vi "Start.vi"(8 "error in (no error)":errorcluster, 10 "Message in":refnum<class "StartMessage.lvclass">, 11 "ImageStack in":refnum<class "Invivo_ImageStack.lvclass">) -> (0 "error out":errorcluster, 3 "ImageStack out":refnum<class "Invivo_ImageStack.lvclass">)   [LabVIEW 2012, in "Invivo_ImageStack.lvclass"]
doc: "This member function is called when the statemachine in the run.vi receives an 'start' command. It relays the message to all observers of the component.\n\nOverride this member function in your derived class if you need additional start functionality (but don't forget to call the parent method)."
uses:
  Invivo_ImageStack.lvclass
  <vilib>/Distrio/Murmex/StartMessage/StartMessage.lvclass
  <vilib>/Distrio/Murmex/StartMessage/run mode enum.ctl
  <vilib>/Distrio/Murmex/GenericMessage/GenericMessage.lvclass
  Invivo_ImageStack.lvclass/Invivo_ImageStack.ctl
  <vilib>/Distrio/Murmex/Murmex/Murmex.lvclass
  <vilib>/Distrio/Murmex/Message/Add or replace parameter.vi
panel:
  # "This member function is called when the statemachine in the run.vi receives an 'start' command. It relays the message to all observers of the component.\n\nOverride this member function in your derived class if you need additional start functionality (but don't forget to call the parent method)."
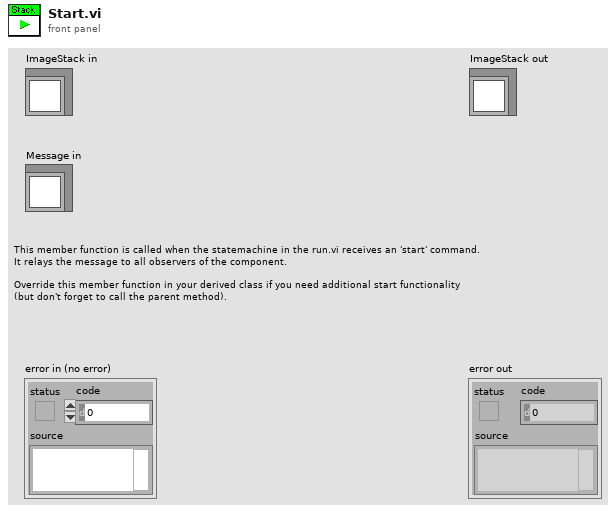
[diagram p1: front panel]
types:
  T1 = typedef "Murmex.lvlib/StartMessage.lvclass/run mode enum.ctl" = enum16{"infinite", "finite"}
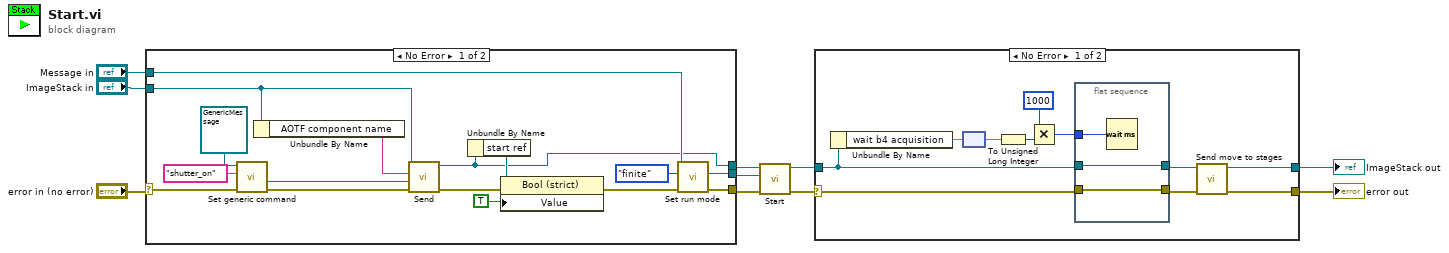
[diagram p0: block diagram]
diagram:
  n1 = case shown="No Error" "error in (no error)" {
    selector: "error in (no error)" -> [w17 w29]
    tunnel: [w25 w29] -> w7
    tunnel: [w18 w28] -> w9
    tunnel: "Message in" -> [w26 w27]
    tunnel: [w23 w27] -> w8
    tunnel: "ImageStack in" -> [w12 w28]
    frame No Error {
      n2 = call <vilib>:"Set generic command.vi"("error in (no error)"=w17, "generic command"="shutter_on", "GenericMessage in"=refnum<class "GenericMessage.lvclass"> refnum ("Distrio Murmex 1.1:GenericMessage")) -> ("error out"=w16:errorcluster, "GenericMessage out"=w13:refnum<class "GenericMessage.lvclass">)  [unwired: 7 in]
      n3 = Unbundle By Name(w12) -> ("AOTF component name"=w11:string)
      n4 = call <vilib>:"Send.vi"("error in (no error)"=w16, "Message"=w13, "recipient"=w11, "Murmex in"=w12) -> ("error out"=w19:errorcluster, "Murmex out"=w18:refnum<class "Invivo_ImageStack.lvclass">)  [unwired: 6 in]
      n5 = Unbundle By Name(w18) -> ("start ref"=w22:refnum<vi>)
      n6 = property class="Bool (strict)"(reference=w22, error in=w19, "Value"=TRUE) -> (error out=w20:errorcluster)  [unwired: 1 out]
      n7 = call <vilib>:"Set run mode.vi"("error in (no error)"=w20, "run mode"=run_mode_enum."finite", "StartMessage in"=w26) -> ("error out"=w25:errorcluster, "StartMessage out"=w23:refnum<class "StartMessage.lvclass">)  [unwired: 7 in]
    }
    frame Error {
    }
  }
  n8 = call-parent "Start.vi"("error in (no error)"=w7, "Message in"=w8, "Murmex in"=w9) -> ("error out"=w4:errorcluster, "Murmex out"=w3:refnum<class "Invivo_ImageStack.lvclass">)  [unwired: 7 in]
  n9 = case shown="No Error" w4 {
    selector: w4 -> [w38 w44]
    tunnel: [w40 w44] -> w1
    tunnel: w3 -> [w35 w45]
    tunnel: [w39 w45] -> w2
    frame No Error {
      n10 = Unbundle By Name(w35) -> ("wait b4 acquisition"=w34:dbl[unit])
      n11 = node(w34) -> (w32:dbl)
      n12 = To Unsigned Long Integer(number=w32) -> (unsigned 32bit integer=w33:u32)
      n13 = Multiply(x=u32 1000, y=w33) -> (x*y=w30:u32)
      n14 = flat-sequence {
        tunnel: w38 -> [w43]
        tunnel: [w43] -> w37
        tunnel: [w42] -> w36
        tunnel: w35 -> [w42]
        tunnel: w30 -> [w41]
        frame #0 {
          n15 = Wait (ms)(milliseconds to wait=w41) -> ()  [unwired: 1 out]
        }
      }
      n16 = call-dynamic "Send move to stages.vi"("error in (no error)"=w37, "ImageStack in"=w36) -> ("error out"=w40:errorcluster, "ImageStack out"=w39:refnum<class "Invivo_ImageStack.lvclass">)  [unwired: 8 in]
    }
    frame Error {
    }
  }
  "error out" <- w1
  "ImageStack out" <- w2
